vi "Sync_time_structs.vi"() -> ()   [LabVIEW 2019]
uses:
  <vilib>/Platform/TimedLoop/XDataNode/timing_clust.ctl
  <vilib>/Platform/TimedLoop/XDataNode/nitl_modes.ctl
  <vilib>/Platform/TimedLoop/XDataNode/wakeup.ctl
  <vilib>/Platform/TimedLoop/scheduler/LVUserAPI/_suppVIs/Create_1kHz_TSource.vi
  <vilib>/platform/TimedLoop/XDataNode/XDataNode.xnode
  <vilib>/Platform/TimedLoop/XDataNode/XDNodeRunTimeDep.lvlib
panel:
  out "Error 2":errorcluster
  out "?":bool
  out "Czas_pocz":u32
  out "Error 1":errorcluster
  out "?":bool
  out "L2 Stop":dbl
  out "L2 End":dbl
  out "Iteracja pêtli L2":dbl
  out "L1 Stop":dbl
  out "L1 End":dbl
  out "Iteracja pêtli L1":dbl
  out "S0 End":dbl
  out "S0 Start":dbl
  in  "Synchronizacja":bool
  in  "Okres pêtli [s]":dbl=0.5 min=0.5 max=20.0 step=0.5
  # "Koniec"
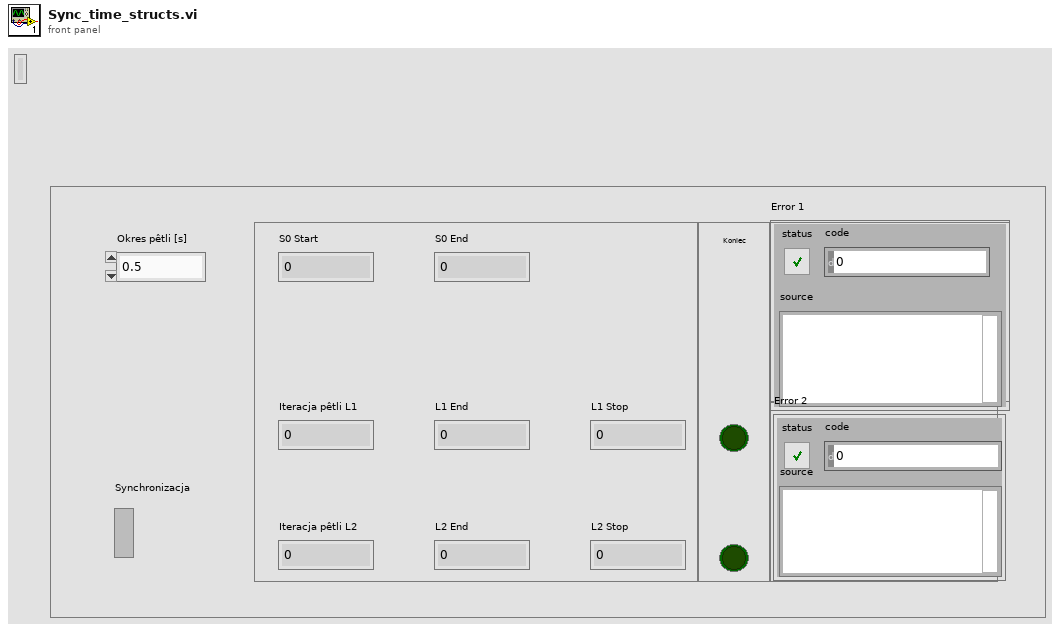
[diagram p1: front panel]
types:
  T1 = typedef "XDNodeRunTimeDep.lvlib/timing_clust.ctl" = cluster{"Expected End [f-1]":u64, "Actual End [f-1]":u64, "Finished Late? [f-1]":bool, "Expected End [i-1]":u64, "Actual End [i-1]":u64, "Finished Late? [i-1]":bool, "Expected Start [i]":u64, "Actual Start [i]":u64, "Expected Start [f]":u64, "Actual Start [f]":u64, "Source Name":string, "Structure Name":string, "Period":i64, "Deadline":i64, "Offset":i64, "Start":i64, "Priority":i32, "Timeout":i32, "Mode":T2, "Wakeup Reason":T3, "Error":errorcluster, "Source Type":string, "Secondary Source Type":string, "Global End Time":u64, "Global Start Time":u64, "Frame Duration":u64, "Iteration Duration":u64, "Assigned CPU":i32, "I/O Scan Engine Mode":u32}
  T2 = typedef "XDNodeRunTimeDep.lvlib/nitl_modes.ctl" = enum32{"No Change", "Process missed periods, maintain original phase", "Discard missed periods, maintain original phase", "Process missed periods, ignore original phase", "Discard missed periods, ignore original phase"}
  T3 = typedef "XDNodeRunTimeDep.lvlib/wakeup.ctl" = enum32{"Normal", "Aborted", "Asynchronous wakeup", "Timing source error", "Timed loop error", "Timeout"}
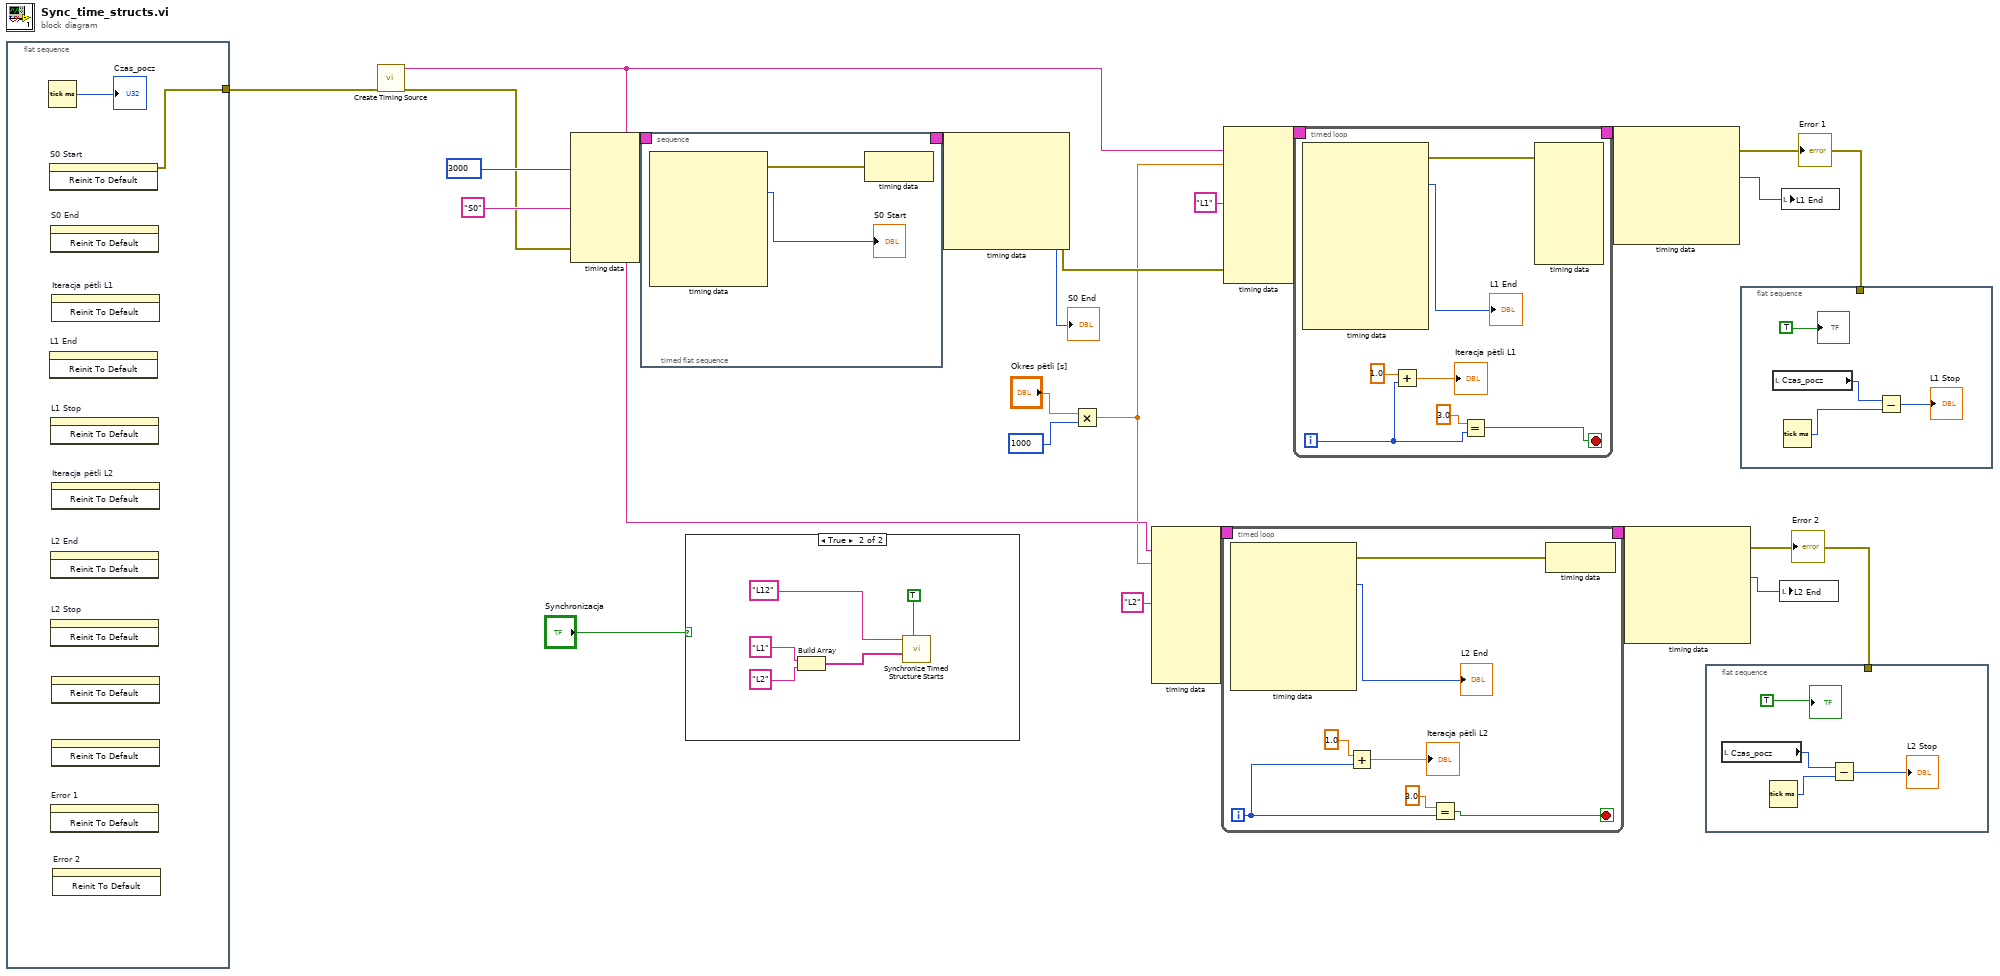
[diagram p0: block diagram]
diagram:
  n1 = flat-sequence {
    tunnel: [w24] -> w2
    frame #0 {
      n2 = Tick Count (ms)() -> (millisecond timer value=→"Czas_pocz":u32)
      n3 = invoke on="S0 Start" class="DigNum (strict)" method="Reinit To Default"() -> (error out=w24:errorcluster)  [unwired: 3 in, 2 out]
      n4 = invoke on="L1 End" class="DigNum (strict)" method="Reinit To Default"() -> ()  [unwired: 3 in, 3 out]
      n5 = invoke on="S0 End" class="DigNum (strict)" method="Reinit To Default"() -> ()  [unwired: 3 in, 3 out]
      n6 = invoke on="L1 Stop" class="DigNum (strict)" method="Reinit To Default"() -> ()  [unwired: 3 in, 3 out]
      n7 = invoke on="L2 End" class="DigNum (strict)" method="Reinit To Default"() -> ()  [unwired: 3 in, 3 out]
      n8 = invoke on="L2 Stop" class="DigNum (strict)" method="Reinit To Default"() -> ()  [unwired: 3 in, 3 out]
      n9 = invoke on="Error 1" class="Clust (strict)" method="Reinit To Default"() -> ()  [unwired: 3 in, 3 out]
      n10 = invoke on="Iteracja pêtli L1" class="DigNum (strict)" method="Reinit To Default"() -> ()  [unwired: 3 in, 3 out]
      n11 = invoke on="Iteracja pêtli L2" class="DigNum (strict)" method="Reinit To Default"() -> ()  [unwired: 3 in, 3 out]
      n12 = invoke class="Bool (strict)" method="Reinit To Default"() -> ()  [unwired: 3 in, 3 out]
      n13 = invoke class="Bool (strict)" method="Reinit To Default"() -> ()  [unwired: 3 in, 3 out]
      n14 = invoke on="Error 2" class="Clust (strict)" method="Reinit To Default"() -> ()  [unwired: 3 in, 3 out]
    }
  }
  n15 = call-poly <vilib>:"Create Timing Source.vi"("error in (no error)"=w2) -> ("error out"=w4:errorcluster, "name (out)"=w14:string)  [unwired: 9 in]
  n16 = node-c288(w14, i64 3000 ("Offset"), "S0" ("Structure Name"), w4) -> (w23:T1)  [unwired: 4 in]
  n17 = timed-sequence {
    timing: w23 -> [_]
    timing-out: [_] -> w22
    n18 = timed-flat-sequence {
      n19 = node-c288() -> (w27:errorcluster, →"S0 Start":i64)  [unwired: 1 in, 7 out]
      n20 = node-c288(w27) -> ()  [unwired: 1 out]
    }
  }
  n21 = case shown="True" "Synchronizacja" {
    frame False {
    }
    frame True {
      n22 = Build Array("L1", "L2") -> (w34:string[])
      n23 = call <vilib>:"Synchronize Timed Structure Starts.vi"("replace (T)"=TRUE, "timed structure names"=w34, "synchronization group name"="L12") -> ()  [unwired: 7 in, 2 out]
    }
  }
  n24 = node-c288(w22) -> (w17:errorcluster, →"S0 End":i64)  [unwired: 5 out]
  n25 = Multiply(x="Okres pêtli [s]", y=1000) -> (x*y=w6:dbl)
  n26 = node-c288(w14, w6, "L2" ("Structure Name")) -> (w19:T1)  [unwired: 7 in]
  n27 = timed-loop {
    timing: w19 -> [_]
    timing-out: [_] -> w18
    i -> [w39]
    stop <- w41 stop-if-true
    n28 = node-c288() -> (w45:errorcluster, →"L2 End":i64)  [unwired: 1 in, 8 out]
    n29 = Add(x=1.0, y=w39) -> (x+y=→"Iteracja pêtli L2":dbl)
    n30 = Equal?(x=3.0, y=w39) -> (x = y?=w41:bool)
    n31 = node-c288(w45) -> ()  [unwired: 1 out]
  }
  n32 = node-c288(w14, w6, "L1" ("Structure Name"), w17) -> (w21:T1)  [unwired: 6 in]
  n33 = timed-loop {
    timing: w21 -> [_]
    timing-out: [_] -> w20
    i -> [w53]
    stop <- w52 stop-if-true
    n34 = node-c288() -> (w58:errorcluster, →"L1 End":i64)  [unwired: 1 in, 11 out]
    n35 = Add(x=1.0, y=w53) -> (x+y=→"Iteracja pêtli L1":dbl)
    n36 = Equal?(x=3.0, y=w53) -> (x = y?=w52:bool)
    n37 = node-c288(w58) -> ()  [unwired: 7 in, 1 out]
  }
  n38 = node-c288(w20) -> (w16:errorcluster, w7:i64)  [unwired: 5 out]
  "Error 1" <- w16
  n39 = node-c288(w18) -> (w15:errorcluster, w5:i64)  [unwired: 5 out]
  "Error 2" <- w15
  n40 = flat-sequence {
    tunnel: w15 -> [_]
    frame #0 {
      n41 = local read "Czas_pocz"() -> (w65:u32)
      n42 = Tick Count (ms)() -> (millisecond timer value=w66:u32)
      n43 = Subtract(x=w65, y=w66) -> (x-y=→"L2 Stop":u32)
      "?" <- TRUE
    }
  }
  n44 = flat-sequence {
    tunnel: w16 -> [_]
    frame #0 {
      n45 = local read "Czas_pocz"() -> (w70:u32)
      n46 = Tick Count (ms)() -> (millisecond timer value=w71:u32)
      n47 = Subtract(x=w70, y=w71) -> (x-y=→"L1 Stop":u32)
      "?" <- TRUE
    }
  }
  n48 = local write "L2 End"(w5) -> ()
  n49 = local write "L1 End"(w7) -> ()
